vi "Disc_select.vi"() -> (0 "Cancel Button 2":bool, 3 "Enum 2":T1)   [LabVIEW 2012]
uses:
  Piezo_Discs.ctl
panel:
  in  "Cancel Button":bool
  in  "OK Button":bool
  in  "Enum":T1
  # "Please select a disc from one of the following options:"
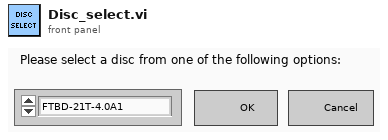
[diagram p1: front panel]
types:
  T1 = typedef "Piezo_Discs.ctl" = enum16{"FTBD-21T-4.0A1", "PZT-5A (Gallas 1)", "PZT-5A (Gallas 2)", "AB4113B", "Create new disc...", "Load disc from file..."}
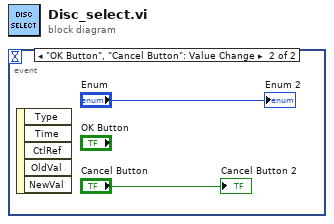
[diagram p0: block diagram]
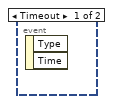
[diagram p2: hidden frame]
diagram:
  n1 = event shown="[1] \"OK Button\", \"Cancel Button\": Value Change" {
    selector: _ -> [_ _]
    dyn-events: _ -> [_ _]
    timeout: _ -> [_ _]
    event Timeout {
      n2 = event-data() -> ()  [unwired: 1 in, 2 out]
    }
    event "OK Button", "Cancel Button": Value Change {
      n3 = event-data() -> ()  [unwired: 1 in, 5 out]
      "Enum 2" <- "Enum"
      "Cancel Button 2" <- "Cancel Button"
    }
  }
